vi "Interpolation.vi"() -> ()   [LabVIEW 2019]
panel:
  in  "X, Y, bool_array 1-line, 0-circle":i32[][](array[numeric])
  out "Y array":i32[](array[numeric])
  out "X array":i32[](array[numeric])
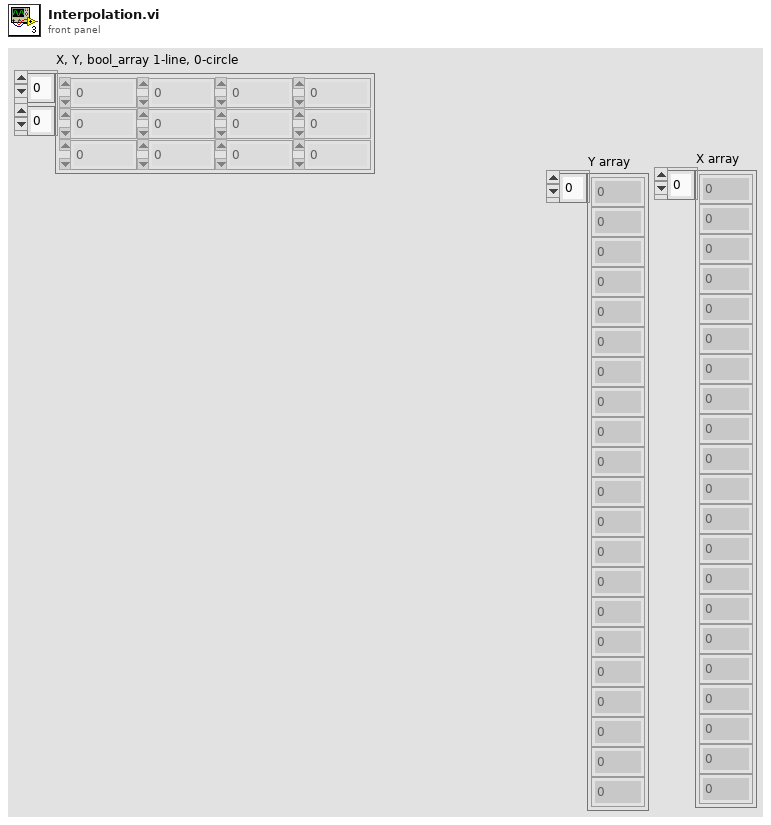
[diagram p1: front panel]
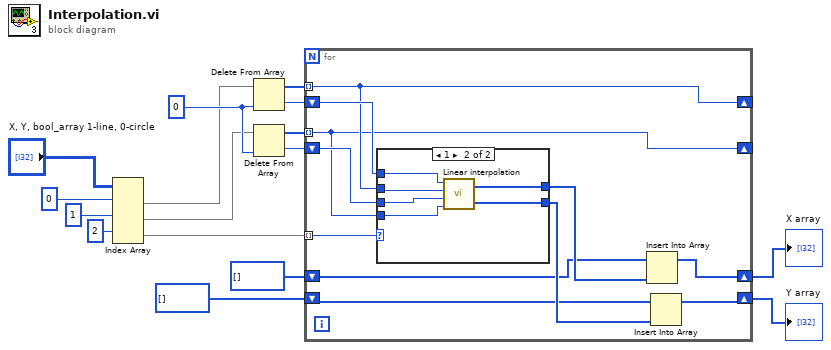
[diagram p0: block diagram]
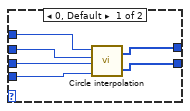
[diagram p2: hidden frame]
diagram:
  w16 = 0 ("index")
  n1 = Index Array(array="X, Y, bool_array 1-line, 0-circle", index (row) #1=0 ("index (row)"), index (row) #2=1 ("index (row)"), index (row) #3=2 ("index (row)")) -> (element #1=w2:i32[], element #2=w1:i32[], element #3=w3:i32[])  [unwired: 3 in]
  n2 = Delete From Array(array=w2, index=w16) -> (deleted portion=w13:i32, array with subset deleted=w14:i32[])  [unwired: 1 in]
  n3 = Delete From Array(array=w1, index=w16) -> (deleted portion=w12:i32, array with subset deleted=w15:i32[])  [unwired: 1 in]
  n4 = for {
    tunnel: w15 -> [w24] mode=indexing
    tunnel: w14 -> [w25] mode=indexing
    shift-right: [w25] -> _
    shift-left: w13 -> [w27]
    shift-right: [w24] -> _
    shift-left: w12 -> [w26]
    shift-right: [w23] -> w8
    shift-left: i32[] [] -> [w20]
    shift-right: [w18] -> w9
    shift-left: i32[] [] -> [w19]
    tunnel: w3 -> [w17] mode=indexing
    n5 = case shown="1" w17 {
      tunnel: w27 -> [w33 w39]
      tunnel: w26 -> [w31 w37]
      tunnel: w25 -> [w32 w38]
      tunnel: w24 -> [w30 w36]
      tunnel: [w29 w35] -> w22
      tunnel: [w28 w34] -> w21
      frame 0, Default {
        n6 = call "Circle interpolation.vi"("Yf"=w30, "Y0"=w31, "Xf"=w32, "X0"=w33) -> ("Y array"=w28:i32[], "X array"=w29:i32[])
      }
      frame 1 {
        n7 = call "Linear interpolation.vi"("Yf"=w36, "Y0"=w37, "Xf"=w38, "X0"=w39) -> ("Y array"=w34:i32[], "X array"=w35:i32[])
      }
    }
    n8 = Insert Into Array(array=w19, new element=w22) -> (w18:i32[])  [unwired: 1 in]
    n9 = Insert Into Array(array=w20, new element=w21) -> (w23:i32[])  [unwired: 1 in]
  }
  "X array" <- w9
  "Y array" <- w8
